vi "Keep Aero Tunnel Seeding on.vi"() -> ()   [LabVIEW 2022 SP3]
panel:
  in  "stop":bool
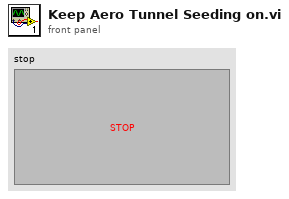
[diagram p1: front panel]
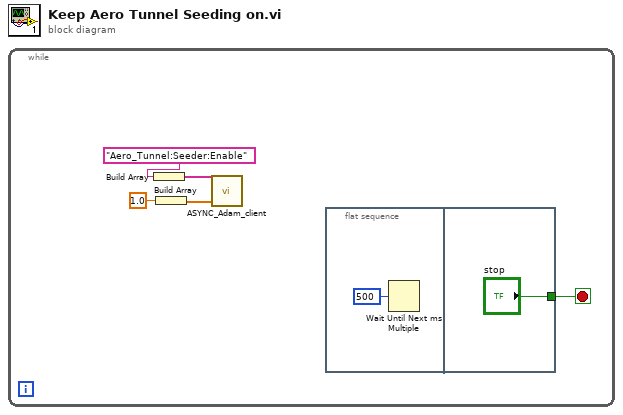
[diagram p0: block diagram]
diagram:
  n1 = while {
    stop <- w1 stop-if-true
    n2 = Build Array("Aero_Tunnel:Seeder:Enable" ("Channel Name")) -> (w5:string[])
    n3 = Build Array(1.0 ("element")) -> (w4:dbl[])
    n4 = call "ASYNC_Adam_client.vi"("Values"=w4, "Channel Names"=w5) -> ()  [unwired: 1 in, 2 out]
    n5 = flat-sequence {
      tunnel: ["stop"] -> w1
      frame #0 {
        n6 = Wait Until Next ms Multiple(millisecond multiple=u32 500 ("milliseconds to wait")) -> ()  [unwired: 1 out]
      }
      frame #1 {
      }
    }
  }
